vi "Joystick Controls to Commands.vi"(11 "Robot Controls":T2) -> (3 "Robot Commands":T1)   [LabVIEW 2014]
uses:
  Robot Control Outputs.ctl
  Robot Commands.ctl
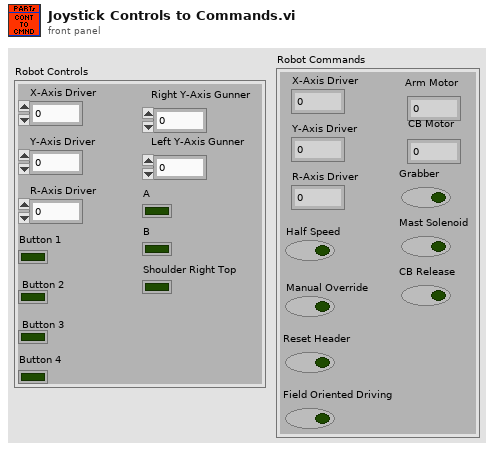
[diagram p1: front panel]
types:
  T1 = typedef "Robot Commands.ctl" = cluster{"X-Axis Driver":dbl, "Y-Axis Driver":dbl, "R-Axis Driver":dbl, "Half Speed":bool, "Manual Override":bool, "Reset Header":bool, "Field Oriented Driving":bool, "Arm Motor":dbl, "CB Motor":dbl, "Grabber":bool, "Mast Solenoid":bool, "CB Release":bool}
  T2 = typedef "Robot Control Outputs.ctl" = cluster{"X-Axis Driver":dbl, "Y-Axis Driver":dbl, "R-Axis Driver":dbl, "Button 1":bool, "Button 2":bool, "Button 3":bool, "Button 4":bool, "Right Y-Axis Gunner":dbl, "Left Y-Axis Gunner":dbl, "A":bool, "B":bool, "Shoulder Right Top ":bool}
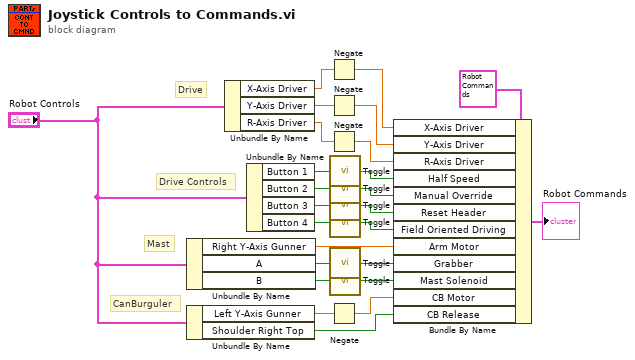
[diagram p0: block diagram]
diagram:
  # "CanBurguler"
  # "Drive Controls"
  # "Mast"
  # "Drive"
  n1 = Unbundle By Name("Robot Controls") -> ("Right Y-Axis Gunner"=w3:dbl, "A"=w17:bool, "B"=w16:bool)
  n2 = Unbundle By Name("Robot Controls") -> ("Left Y-Axis Gunner"=w18:dbl, "Shoulder Right Top"=w7:bool)
  n3 = Unbundle By Name("Robot Controls") -> ("X-Axis Driver"=w25:dbl, "Y-Axis Driver"=w24:dbl, "R-Axis Driver"=w23:dbl)
  n4 = Unbundle By Name("Robot Controls") -> ("Button 1"=w22:bool, "Button 2"=w21:bool, "Button 3"=w20:bool, "Button 4"=w2:bool)
  n5 = Negate(x=w25) -> (-x=w13:dbl)
  n6 = Negate(x=w24) -> (-x=w12:dbl)
  n7 = Negate(x=w23) -> (-x=w11:dbl)
  n8 = Negate(x=w18) -> (-x=w6:dbl)
  n9 = call "Toggle.vi"("Input"=w22) -> ("Output"=w10:bool)  [unwired: 4 in]
  n10 = call "Toggle.vi"("Input"=w21) -> ("Output"=w9:bool)  [unwired: 4 in]
  n11 = call "Toggle.vi"("Input"=w20) -> ("Output"=w8:bool)  [unwired: 4 in]
  n12 = call "Toggle.vi"("Input"=w2) -> ("Output"=w1:bool)  [unwired: 4 in]
  n13 = call "Toggle.vi"("Input"=w17) -> ("Output"=w4:bool)  [unwired: 4 in]
  n14 = call "Toggle.vi"("Input"=w16) -> ("Output"=w5:bool)  [unwired: 4 in]
  n15 = Bundle By Name(cluster=T1 {"X-Axis Driver"=0.0, "Y-Axis Driver"=0.0, "R-Axis Driver"=0.0, "Half Speed"=FALSE, "Manual Override"=FALSE, "Reset Header"=FALSE, "Field Oriented Driving"=FALSE, "Arm Motor"=0.0, "CB Motor"=0.0, "Grabber"=FALSE, "Mast Solenoid"=FALSE, "CB Release"=FALSE} ("Robot Controls"), "X-Axis Driver"=w13, "Y-Axis Driver"=w12, "R-Axis Driver"=w11, "Half Speed"=w10, "Manual Override"=w9, "Reset Header"=w8, "Field Oriented Driving"=w1, "Arm Motor"=w3, "Grabber"=w4, "Mast Solenoid"=w5, "CB Motor"=w6, "CB Release"=w7) -> (→"Robot Commands":T1)
